vi "Init.vi"(3 "Container State":T3, 4 "Previous State":variant, 5 "Previous Version":T2) -> (2 "Current State":T1)   [LabVIEW 2024, in "Twinkle Button.xctl"]
doc: "本VI是为《我和LabVIEW》一书编写的示例。\n关于本书的介绍请参考网页：\nhttp://ruanqizhen.spaces.live.com/blog/cns!5852D4F797C53FB6!4310.entry"
uses:
  Twinkle Button.xctl
  State.ctl
  <resource>/importtools/Common/Event/NISAST Event.lvclass
  <vilib>/_xctls/Container State.ctl
  <vilib>/_xctls/Version.ctl
  <vilib>/_xctls/XControlSupport.lvlib
panel:
  in  "Default Indicator State":T1
  in  "Default Control State":T1
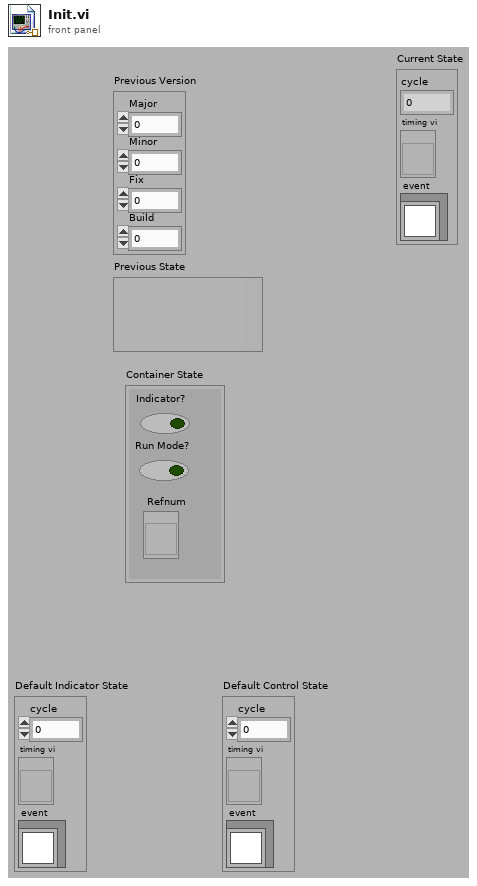
[diagram p1: front panel]
types:
  T1 = typedef "Twinkle Button.xctl/State.ctl" = cluster{"cycle":dbl, "timing vi":refnum<vi>, "event":refnum<class "NISAST Event.lvclass">}
  T2 = typedef "XControlSupport.lvlib/Version.ctl" = cluster{"Major":u16, "Minor":u16, "Fix":u16, "Build":u16}
  T3 = typedef "XControlSupport.lvlib/Container State.ctl" = cluster{"Indicator?":bool, "Run Mode?":bool, " Refnum":refnum<vi>}
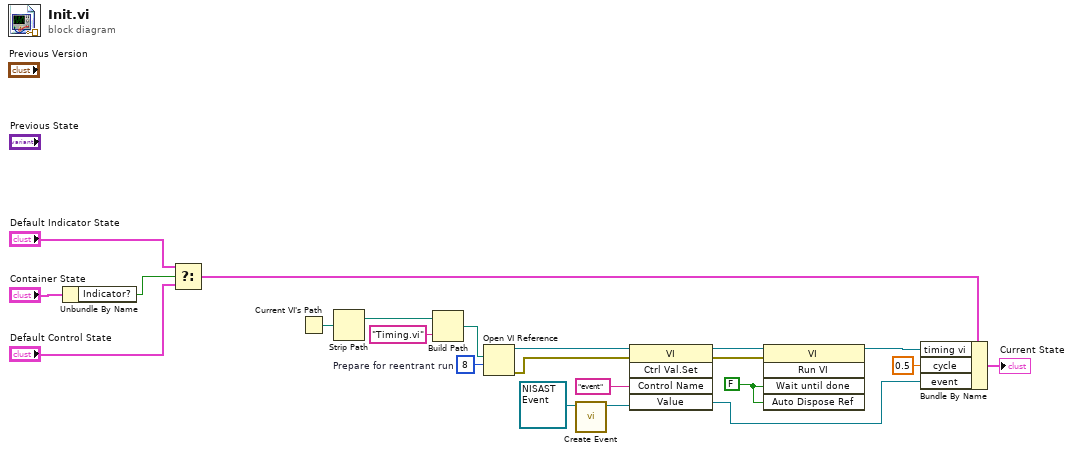
[diagram p0: block diagram]
diagram:
  w10 = FALSE ("Wait Until Done")
  w2 = 8  # Prepare for reentrant run
  n1 = Unbundle By Name("Container State") -> ("Indicator?"=w18:bool)
  n2 = Select(t="Default Indicator State", s=w18, f="Default Control State") -> (s? t:f=w17:T1)
  n3 = Current VI's Path() -> (path=w15:path)
  n4 = Strip Path(path=w15) -> (stripped path=w14:path)  [unwired: 1 out]
  n5 = Build Path(base path=w14, name or relative path="Timing.vi") -> (appended path=w12:path)
  n6 = Open VI Reference(vi path=w12, options=w2) -> (vi reference=w6:refnum<vi>, error out=w5:errorcluster)  [unwired: 1 in, 3 out]
  n7 = call-dynamic "Create Event.vi"("Event in"=refnum<class "NISAST Event.lvclass"> refnum) -> ("Event out"=w3:refnum<class "NISAST Event.lvclass">)  [unwired: 1 in, 9 out]
  n8 = invoke class="VI" method="Ctrl Val.Set"(reference=w6, error in=w5, "Control Name"="event", "Value"=w3) -> (reference out=w8:refnum<vi>, error out=w9:errorcluster)  [unwired: 1 in, 3 out]
  n9 = invoke class="VI" method="Run VI"(reference=w8, error in=w9, "Wait until done"=w10, "Auto Dispose Ref"=w10) -> (reference out=w4:refnum<vi>)  [unwired: 1 in, 4 out]
  n10 = Bundle By Name(cluster=w17, "timing vi"=w4, "cycle"=0.5, "event"=w3) -> (→"Current State":T1)
